vi "Write Tmirror.vi"(8 "error in (no error)":errorcluster, 10 "Tmirror":dbl, 11 "CR5 Data in":refnum<class "CR5 Data.lvclass">) -> (0 "error out":errorcluster, 3 "CR5 Data out":refnum<class "CR5 Data.lvclass">)   [LabVIEW 2015, in "CR5 Data.lvclass"]
uses:
  CR5 Data.lvclass
  CR5 Data.lvclass/CR5 Data.ctl
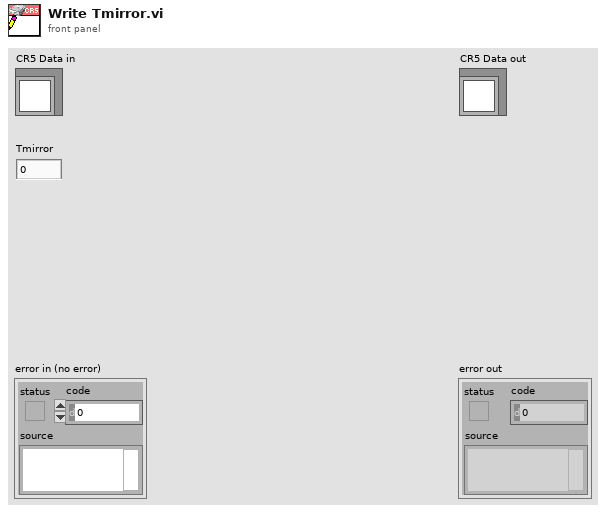
[diagram p1: front panel]
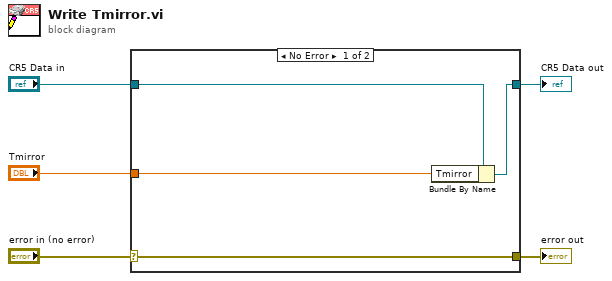
[diagram p0: block diagram]
diagram:
  n1 = case shown="No Error" "error in (no error)" {
    selector: "error in (no error)" -> [w9 w10]
    tunnel: [w9 w10] -> w4
    tunnel: [w7 w11] -> w2
    tunnel: "CR5 Data in" -> [w8 w11]
    tunnel: "Tmirror" -> [w6 _]
    frame No Error {
      n2 = Bundle By Name(cluster=w8, "Tmirror"=w6) -> (w7:refnum<class "CR5 Data.lvclass">)
    }
    frame Error {
    }
  }
  "error out" <- w4
  "CR5 Data out" <- w2
